vi "FTW-TransferClient-PostEvent-Progress.vi"(4 "TotalBytes":i64, 5 "Timestamp":u32, 6 "TransferredBytes":i64, 7 "Initial Timestamp":u32, 8 "Percent Done":i32, 9 "Local Filepath":path, 10 "Remote URI":string, 11 "Transfer Progress Event":refnum<user-event>) -> ()   [LabVIEW 2012, in "FTW-TransferClient.lvclass"]
uses:
  FTW-TransferClient.lvclass
  FTW-TransferClient-TransferProgress.ctl
  Core/src/Numeric/FTW-NUM-MovingAverage.vi
  Core/src/Time/FTW-Time-Elapse.vi
panel:
  # "Inputs"
  # "Outputs"
  # "No Outputs - this VI\nis fire and forget"
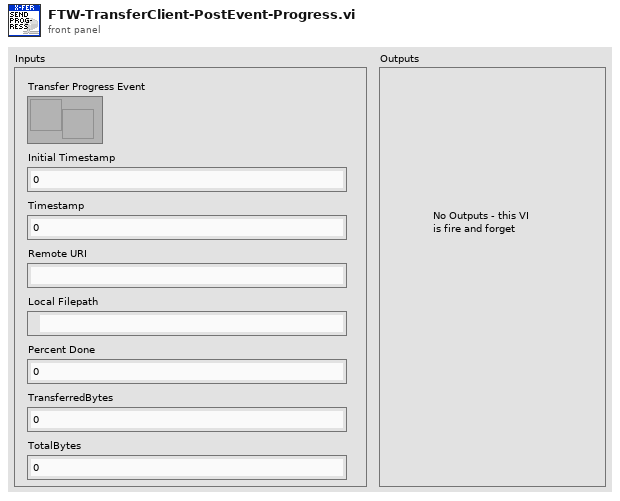
[diagram p1: front panel]
types:
  T1 = typedef "FTW-TransferClient-TransferProgress.ctl" = cluster{"Remote URI":string, "Local Filepath":path, "Total Bytes":i64, "Transferred Bytes":i64, "Percent Complete":dbl, "Current Rate":dbl, "Time Elapsed":u32, "Est. Time Remaining":u32}
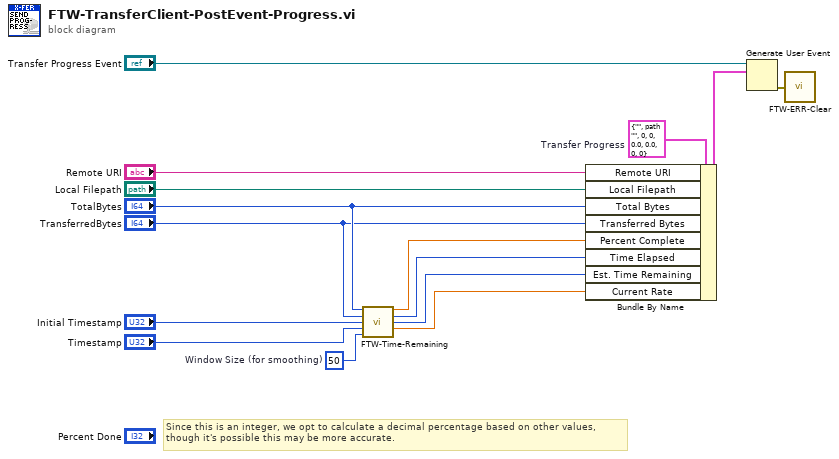
[diagram p0: block diagram]
diagram:
  w3 = 50  # Window Size (for smoothing)
  w12 = T1 {"Remote URI"="", "Local Filepath"=path "", "Total Bytes"=0, "Transferred Bytes"=0, "Percent Complete"=0.0, "Current Rate"=0.0, "Time Elapsed"=0, "Est. Time Remaining"=0}  # Transfer Progress
  # "Since this is an integer, we opt to calculate a decimal percentage based on other values,\nthough it's possible this may be more accurate."
  n1 = call "FTW-Time-Remaining.vi"("Total Work Units"="TotalBytes", "Work Units Complete"="TransferredBytes", "Initial Timestamp"="Initial Timestamp", "Current Timestamp"="Timestamp", "Window Size (for smoothing)"=w3) -> ("Percent Done (0.0-100.0%)"=w8:dbl, "Time Elapsed (msec)"=w9:u32, "Estimated Time Remaining (msec)"=w1:u32, "Current Rate (Units of Work per sec)"=w2:dbl)  [unwired: 6 in, 1 out]
  n2 = Bundle By Name(cluster=w12, "Remote URI"="Remote URI", "Local Filepath"="Local Filepath", "Total Bytes"="TotalBytes", "Transferred Bytes"="TransferredBytes", "Percent Complete"=w8, "Time Elapsed"=w9, "Est. Time Remaining"=w1, "Current Rate"=w2) -> (w15:T1)
  n3 = Generate User Event(user event="Transfer Progress Event", event data cluster=w15) -> (error out=w10:errorcluster)  [unwired: 1 in, 1 out]
  n4 = call "FTW-ERR-Clear.vi"("error to snuff"=w10) -> ()  [unwired: 1 out]
